vi "AP Position.vi"(1 "Coordinates":dbl[][](array[numeric]) format="%.6f") -> (0 "AP Position":T1)   [LabVIEW 2010]
uses:
  <vilib>/Analysis/baseanly.llb/A x Vector.vi
  <vilib>/Analysis/NI_AALBase.lvlib
panel:
  out "[R]T Trunk":dbl[][](array[numeric])
  out "[R] Trunk":dbl[][](array[numeric])
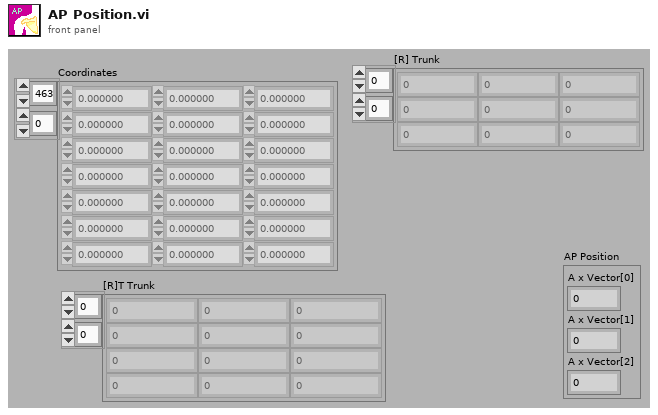
[diagram p1: front panel]
types:
  T1 = cluster{"A x Vector[0]":dbl, "A x Vector[1]":dbl, "A x Vector[2]":dbl}
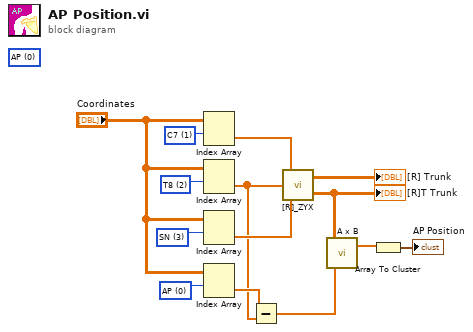
[diagram p0: block diagram]
diagram:
  w13 = u16 3 items=["AP", "C7", "T8", "SN", "XP", "LM", "MM", "WR"] ("Marker Names")
  w9 = u16 1 items=["AP", "C7", "T8", "SN", "XP", "LM", "MM", "WR"] ("Marker Names")
  w8 = u16 2 items=["AP", "C7", "T8", "SN", "XP", "LM", "MM", "WR"] ("Marker Names")
  w14 = u16 0 items=["AP", "C7", "T8", "SN", "XP", "LM", "MM", "WR"] ("Marker Names")
  (unwired) u16 0 items=["AP", "C7", "T8", "SN", "XP", "LM", "MM", "WR"] ("Marker Names")
  n1 = Index Array(array="Coordinates", index (row)=w9) -> (element=w12:dbl[])  [unwired: 1 in]
  n2 = Index Array(array="Coordinates", index (row)=w8) -> (element=w2:dbl[])  [unwired: 1 in]
  n3 = Index Array(array="Coordinates", index (row)=w13) -> (element=w11:dbl[])  [unwired: 1 in]
  n4 = Index Array(array="Coordinates", index (row)=w14) -> (element=w3:dbl[])  [unwired: 1 in]
  n5 = Subtract(x=w3, y=w2) -> (x-y=w1:dbl[])
  n6 = call "[R]_ZYX.vi"("Marker 2"=w11, "Origin"=w2, "Marker 1"=w12) -> ("[R]T"=w5:dbl[][], "[R]"=→"[R] Trunk":dbl[][])
  "[R]T Trunk" <- w5
  n7 = call-poly <vilib>:"A x B.vi"("Vector"=w1, "A"=w5) -> ("A x Vector"=w4:dbl[])  [unwired: 1 out]
  n8 = Array To Cluster(array=w4) -> (cluster=→"AP Position":T1)
